vi "Cap_TRJ.vi"(0 "Element Description":string, 1 "Measured origin x,y":dbl[](array[numeric])=[0.83, 0.79], 2 "Additional Stuff":i32, 3 "Mode":u16(ring) items=["Get Path", "Write Files"]) -> (4 "Start Point":dbl[][](array[numeric]), 5 "trj file path":path[](array[path]), 6 "path":path, 7 "size(s)":i32, 8 "XY Line Arc Trajectory":T1={"Velocity (units/s)"=2.0, "Acceleration (unts/s2)"=20.0, "Number of times of execution"=1} {"Acceleration (unts/s2)" format="%.6f"; "Velocity (units/s)" format="%.6f"; "Number of times of execution" format="%.6f"})   [LabVIEW 2009]
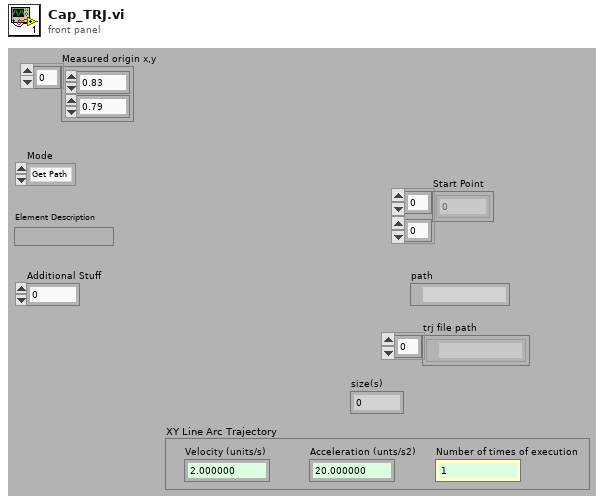
[diagram p1: front panel]
types:
  T1 = cluster{"Velocity (units/s)":dbl, "Acceleration (unts/s2)":dbl, "Number of times of execution":i32}
  T2 = cluster{"delimiter (Tab)":dbl, "delimiter (Tab)":dbl, "delimiter (Tab)":dbl}
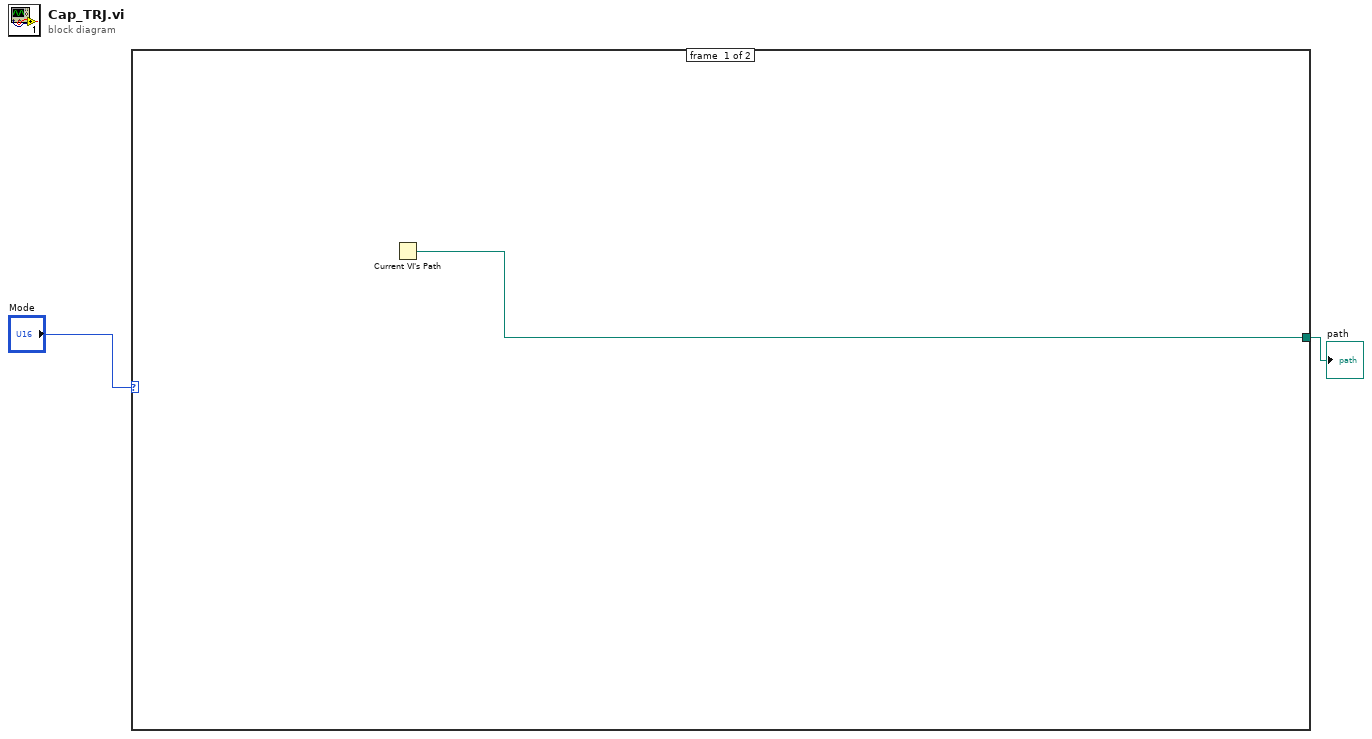
[diagram p0: block diagram]
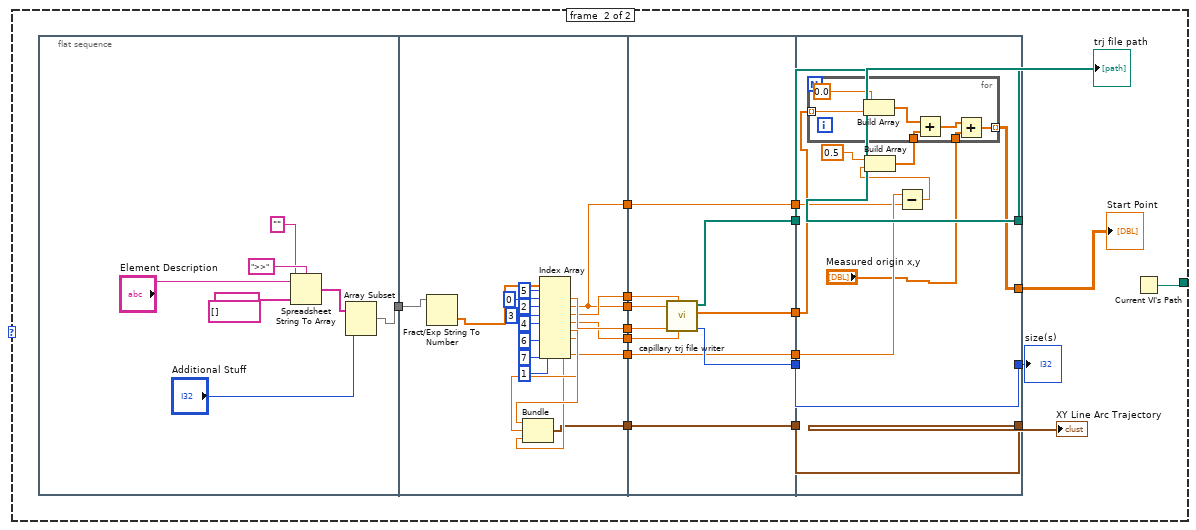
[diagram p2: hidden frame]
diagram:
  n1 = case shown="1" "Mode" {
    tunnel: [w3 w13] -> w1
    frame #0 {
      n2 = Current VI's Path() -> (path=w3:path)
    }
    frame #1 {
      n3 = flat-sequence {
        tunnel: [w24] -> w22
        tunnel: w22 -> [w48]
        tunnel: [w45] -> w21
        tunnel: [w30] -> w20
        tunnel: [w42] -> w19
        tunnel: [w40] -> w18
        tunnel: [w33] -> w17
        tunnel: [w31] -> w7
        tunnel: [w30] -> w5
        tunnel: w21 -> [w58]
        tunnel: w20 -> [w57]
        tunnel: w19 -> [w56]
        tunnel: w18 -> [w55]
        tunnel: w17 -> [w54]
        tunnel: [w54] -> w12
        tunnel: [w53] -> w11
        tunnel: [w52] -> w10
        tunnel: [w51] -> w9
        tunnel: [w50] -> w8
        tunnel: w7 -> [w50]
        tunnel: [w49] -> w6
        tunnel: w5 -> [w49]
        tunnel: [w67] -> w15
        tunnel: [w68] -> w14
        tunnel: [w69] -> w16
        tunnel: w12 -> [w69]
        tunnel: w11 -> [w68]
        tunnel: w10 -> [w61]
        tunnel: w9 -> [w67]
        tunnel: w8 -> [w66]
        tunnel: w6 -> [w65]
        tunnel: [w60] -> w4
        frame #0 {
          n4 = Spreadsheet String To Array(delimiter (Tab)=">>", format string="" ("delimiter (Tab)"), spreadsheet string="Element Description", array type (2D Dbl)=string[] []) -> (array=w25:string[])
          n5 = Array Subset(array=w25, index="Additional Stuff") -> (w24:string[])  [unwired: 1 in]
        }
        frame #1 {
          n6 = Fract/Exp String To Number(string=w48) -> (number=w47:dbl[])  [unwired: 3 in, 1 out]
          n7 = Index Array(array=w47, index #1=0 ("index"), index #2=2 ("index"), index #3=3 ("index"), index #4=4 ("index"), index #5=5 ("index"), index #6=6 ("index"), index #7=7 ("index"), index #8=1 ("index")) -> (element #1=w45:dbl, element #2=w30:dbl, element #3=w42:dbl, element #4=w40:dbl, element #5=w36:dbl, element #6=w35:dbl, element #7=w34:dbl, element #8=w31:dbl)
          n8 = Bundle("delimiter (Tab)"=w36, "delimiter (Tab)"=w35, "delimiter (Tab)"=w34) -> (w33:T2)  [unwired: 1 in]
        }
        frame #2 {
          n9 = call "capillary trj file writer.vi"("interval between laser path"=w55, "ablation rate"=w56, "length of capillary"=w58, "radus of cap"=w57) -> ("size(s)"=w51:i32, "start point"=w52:dbl[], "trj file path(1)"=w53:path[])  [unwired: 3 out]
        }
        frame #3 {
          n10 = Subtract(x=w66, y=w65) -> (x-y=w62:dbl)
          n11 = Build Array(0.5 ("element"), w62) -> (w64:dbl[])
          n12 = for {
            tunnel: w64 -> [w75]
            tunnel: "Measured origin x,y" -> [w72]
            tunnel: w61 -> [w71] mode=indexing
            tunnel: [w70] -> w60 mode=indexing
            n13 = Build Array(0.0 ("element"), w71) -> (w74:dbl[])
            n14 = Add(x=w74, y=w75) -> (x+y=w76:dbl[])
            n15 = Add(x=w76, y=w72) -> (x+y=w70:dbl[])
          }
        }
      }
      n16 = Current VI's Path() -> (path=w13:path)
      "XY Line Arc Trajectory" <- w16
      "size(s)" <- w15
      "trj file path" <- w14
      "Start Point" <- w4
    }
  }
  "path" <- w1
